vi "DSF.Execution.Runtime.Plugin Manager.Load Plugins.vi"(8 "error in (no error)":errorcluster, 10 "Plugin names":string[](array[string]), 11 "Plugin Manager in":refnum<class "DSF.Engine.Runtime.Plugin Manager.lvclass">) -> (0 "error out":errorcluster, 2 "Plugins":refnum<class "Plugin.lvclass">[](array[class]), 3 "Plugin Manager out":refnum<class "DSF.Engine.Runtime.Plugin Manager.lvclass">)   [LabVIEW 2016, in "DSF.Engine.lvlib" / "DSF.Engine.Runtime.Plugin Manager.lvclass"]
uses:
  DSF.Engine.Runtime.Plugin Manager.lvclass
  Plugin/Plugin.lvclass
  DSF.Engine.Runtime.Plugin Manager.lvclass/DSF.Engine.Runtime.Plugin Manager.ctl
  DSF.Execution.Runtime.Plugin Manager.Objects to Plugin.vi
  DSF.Execution.Runtime.Plugin Manager.Query Disk.Classes.Plugin.vi
  DSF.Execution.Runtime.Plugin Manager.Load Classes.vi
  DSF.Execution.Runtime.Plugin Manager.Load Plugin Classes.Configuration.vi
  DSF.Execution.Runtime.Plugin Manager.Load Plugin Classes.Runtime.vi
  DSF.Execution.Runtime.Plugin Manager.Query Disk.Classes.vi
  DSF.Execution.Runtime.Plugin Manager.Name to Path.vi
  DSF.Execution.Runtime.Plugin Manager.Get Plugins Folder.vi
  Plugin/DSF.Engine.Plugin.Initialize.vi
  Shared/Classes/Plugin/DSF.Shared.Runtime.Plugin.Find First Instance.vi
  Shared/Classes/Transfer/DSF.Shared.Configuration.Transfer.Find First Instance.vi
  Shared/Classes/Transfer Group/DSF.Shared.Configuration.Transfer Group.Find First Instance.vi
  Shared/Classes/Plugin/DSF.Shared.Configuration.Plugin.Find First Instance.vi
  <vilib>/Utility/LVClass/Get LV Class Default Value.vi
  <vilib>/Utility/libraryn.llb/Check if File or Folder Exists.vi
  <vilib>/Utility/libraryn.llb/Recursive File List.vi
  Plugin/DSF.Engine.Runtime.Plugin.lvclass
  Shared/Classes/Plugin/DSF.Shared.Configuration.Plugin.lvclass
  Shared/Classes/Transfer Group/DSF.Shared.Configuration.Transfer Group.lvclass
  Shared/Classes/Transfer/DSF.Shared.Configuration.Transfer.lvclass
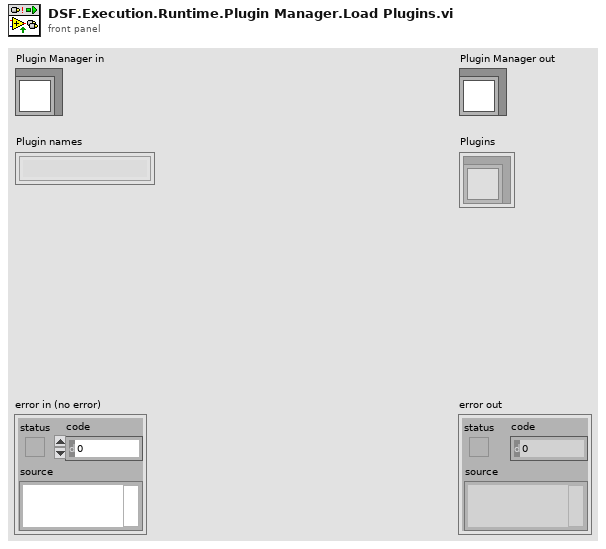
[diagram p1: front panel]
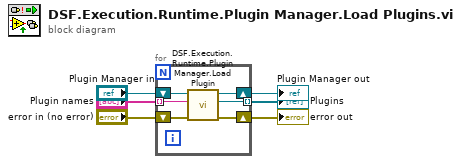
[diagram p0: block diagram]
diagram:
  n1 = for {
    tunnel: "Plugin names" -> [w11] mode=indexing
    shift-right: [w9] -> w2
    shift-left: "Plugin Manager in" -> [w12]
    shift-right: [w8] -> w1
    shift-left: "error in (no error)" -> [w10]
    tunnel: [w7] -> w3 mode=indexing
    n2 = call "DSF.Execution.Runtime.Plugin Manager.Load Plugin.vi"("error in (no error)"=w10, "Plugin name"=w11, "Plugin Manager in"=w12) -> ("error out"=w8:errorcluster, "Plugin"=w7:refnum<class "Plugin.lvclass">, "Plugin Manager out"=w9:refnum<class "DSF.Engine.Runtime.Plugin Manager.lvclass">)  [unwired: 6 in]
  }
  "error out" <- w1
  "Plugin Manager out" <- w2
  "Plugins" <- w3
